vi "termoap.vi"() -> ()   [LabVIEW 2020]
uses:
  <vilib>/Instr/_visa.llb/VISA Configure Serial Port (Instr).vi
panel:
  out "mV":i32 format="%#.1f"
  out "mV":dbl(knob) scale=0.0..5000.0
  out "Faren":i32 format="%#.1f"
  out "Faren T":dbl(slide) scale=32.0..1875.2
  out "Rankine":i32 format="%#.1f"
  out "Rankine T":dbl(slide) scale=491.67..2334.87
  out "Kelvin":i32 format="%#.1f"
  out "Kelvin 2":dbl(slide) scale=1297.15..1426.865
  out "Grados":i32 format="%#.1f"
  out "Celsius":dbl(slide) scale=0.0..1024.0
  in  "stop":bool
  in  "VISA resource name":refnum<visa-resource-name>
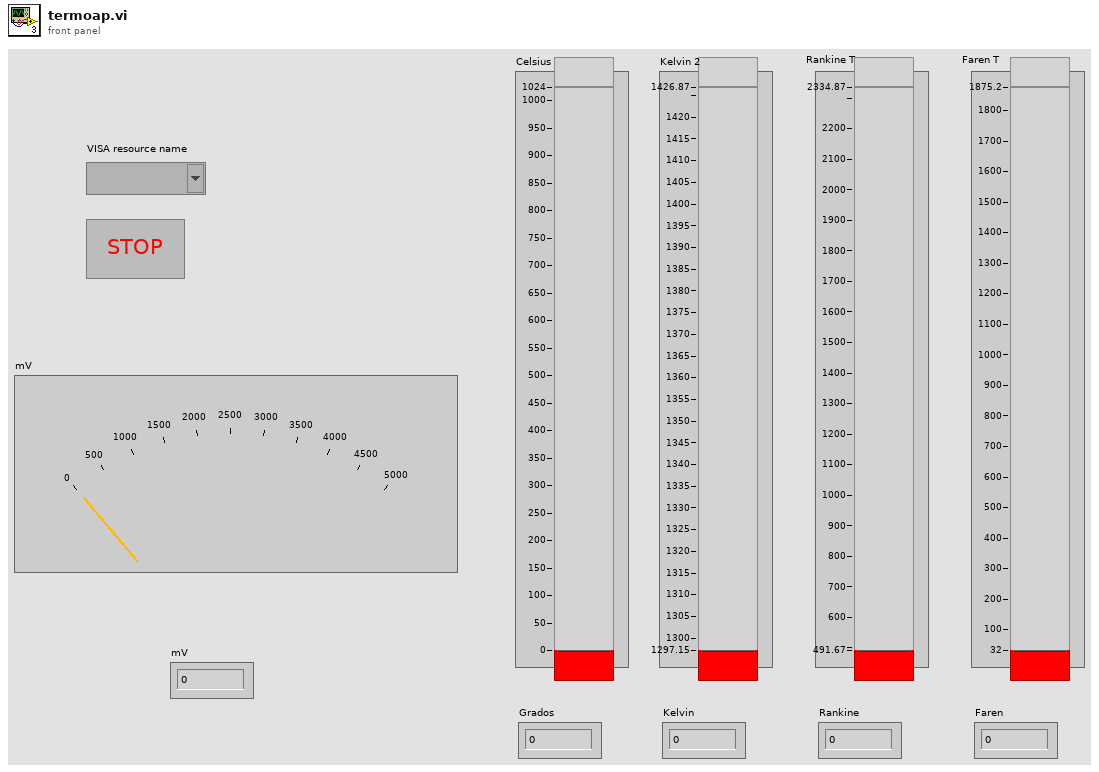
[diagram p1: front panel]
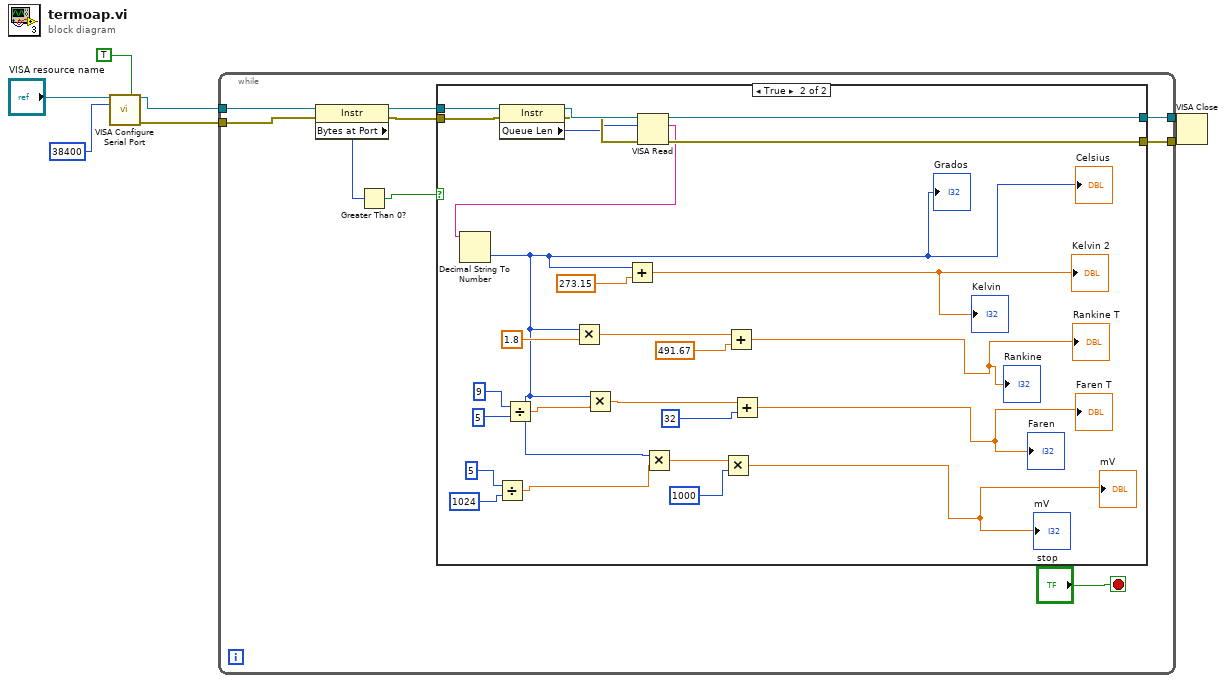
[diagram p0: block diagram]
diagram:
  n1 = call-poly "VISA Configure Serial Port"("VISA resource name"="VISA resource name", "Enable Termination\nChar (T)"=TRUE ("Enable Termination\nChar (T)"), "baud rate (9600)"=u32 38400) -> ("VISA resource name out"=w4:refnum<visa-resource-name>, "error out"=w3:errorcluster)  [unwired: 11 in]
  n2 = while {
    tunnel: w4 -> [w15]
    tunnel: w3 -> [w13]
    tunnel: [w10] -> w2
    tunnel: [w9] -> w1
    stop <- "stop" stop-if-true
    n3 = property class="Instr"(reference=w15, error in=w13) -> (reference out=w14:refnum<visa-resource-name>, error out=w12:errorcluster, "Bytes at Port"=w11:u32)
    n4 = Greater Than 0?(x=w11) -> (x > 0?=w16:bool)
    n5 = case shown="True" w16 {
      tunnel: w14 -> [w18 w45]
      tunnel: w12 -> [w17 w44]
      tunnel: [w18 w41] -> w10
      tunnel: [w17 w40] -> w9
      frame False {
      }
      frame True {
        n6 = Divide(x=5, y=1024) -> (x/y=w27:dbl)
        n7 = property class="Instr"(reference=w45, error in=w44) -> (reference out=w43:refnum<visa-resource-name>, error out=w42:errorcluster, "Queue Len"=w39:u32)
        n8 = Divide(x=9, y=5) -> (x/y=w29:dbl)
        n9 = VISA Read(VISA resource name=w43, byte count=w39, error in (no error)=w42) -> (VISA resource name out=w41:refnum<visa-resource-name>, read buffer=w38:string, error out=w40:errorcluster)  [unwired: 1 out]
        n10 = Decimal String To Number(string=w38) -> (number=w23:i32)  [unwired: 2 in, 1 out]
        "Celsius" <- w23
        "Grados" <- w23
        n11 = Multiply(x=w23, y=1.8) -> (x*y=w34:dbl)
        n12 = Multiply(x=w23, y=w29) -> (x*y=w30:dbl)
        n13 = Add(x=w23, y=273.15) -> (x+y=→"Kelvin 2" →"Kelvin":dbl)
        n14 = Multiply(x=w23, y=w27) -> (x*y=w26:dbl)
        n15 = Multiply(x=w26, y=1000) -> (x*y=→"mV" →"mV":dbl)
        n16 = Add(x=w34, y=491.67) -> (x+y=→"Rankine T" →"Rankine":dbl)
        n17 = Add(x=w30, y=32) -> (x+y=→"Faren T" →"Faren":dbl)
      }
    }
  }
  n18 = VISA Close(VISA resource name=w2, error in (no error)=w1) -> ()  [unwired: 1 out]
